vi "walidacjaTestow.vi"(11 "Odleglosci":T1[][](array[typedef]) {"Odległość [m]" format="%#.2g"}) -> (3 "Testy przeszły?":bool)   [LabVIEW 2014]
uses:
  testujPunktyVIs/Odleglosc.ctl
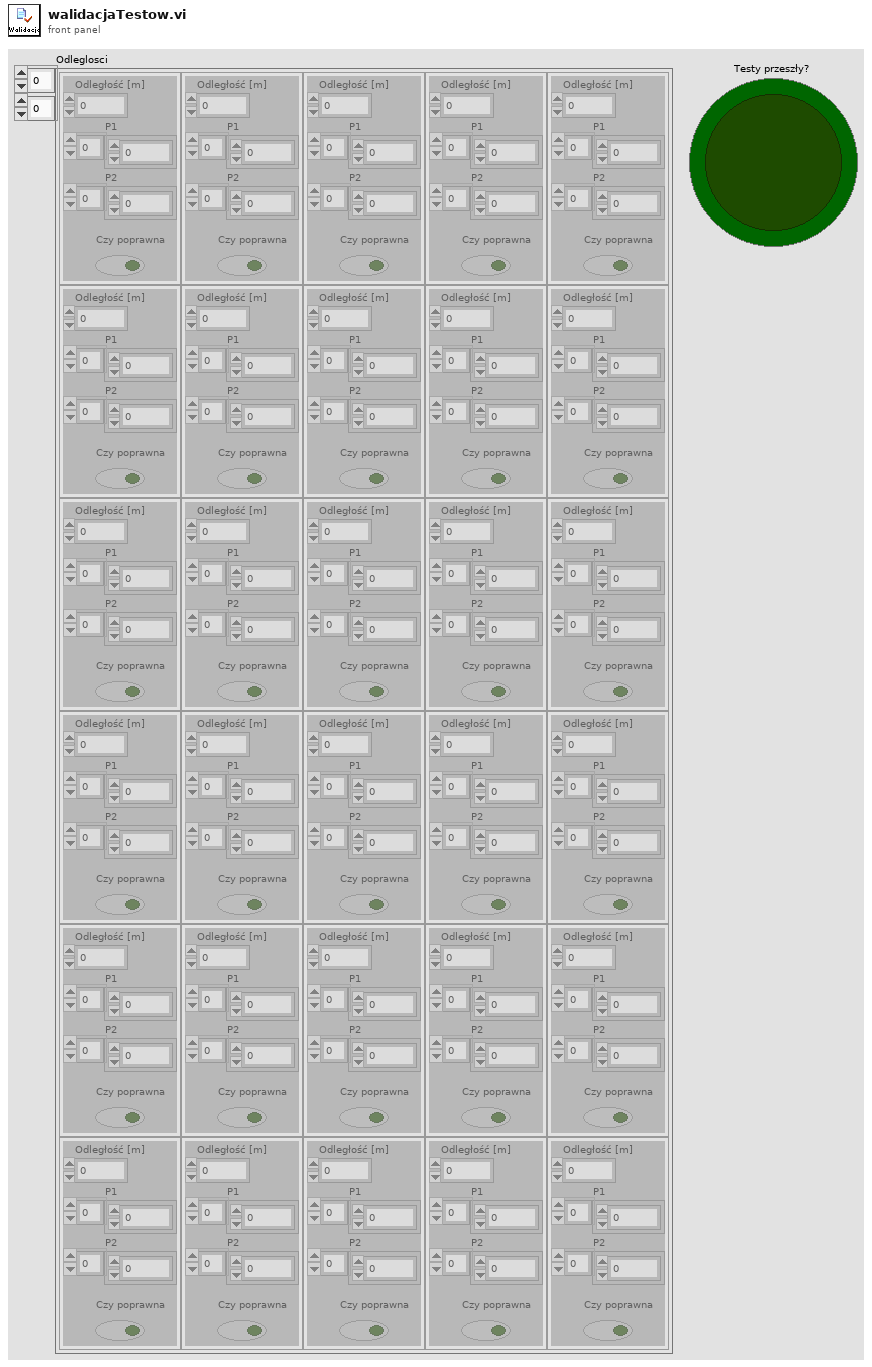
[diagram p1: front panel]
types:
  T1 = typedef "Odleglosc.ctl" = cluster{"Odległość [m]":dbl, "P1":i32[], "P2":i32[], "Czy poprawna":bool}
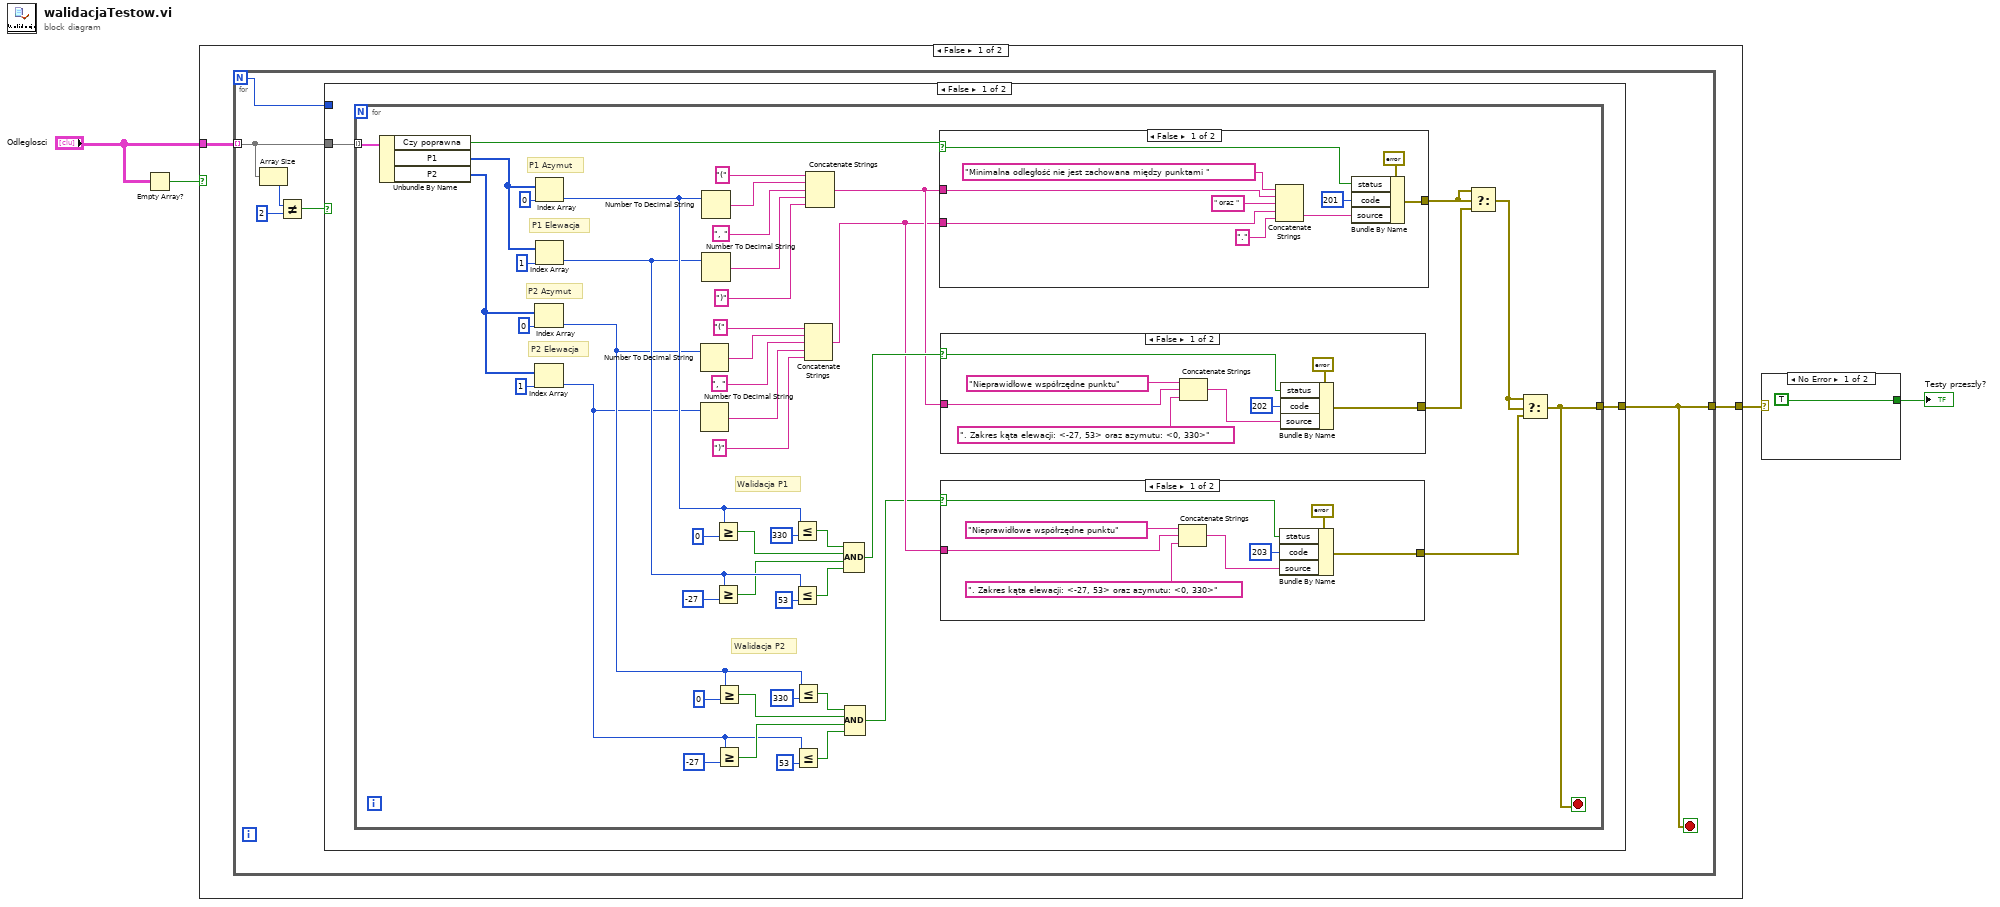
[diagram p0: block diagram]
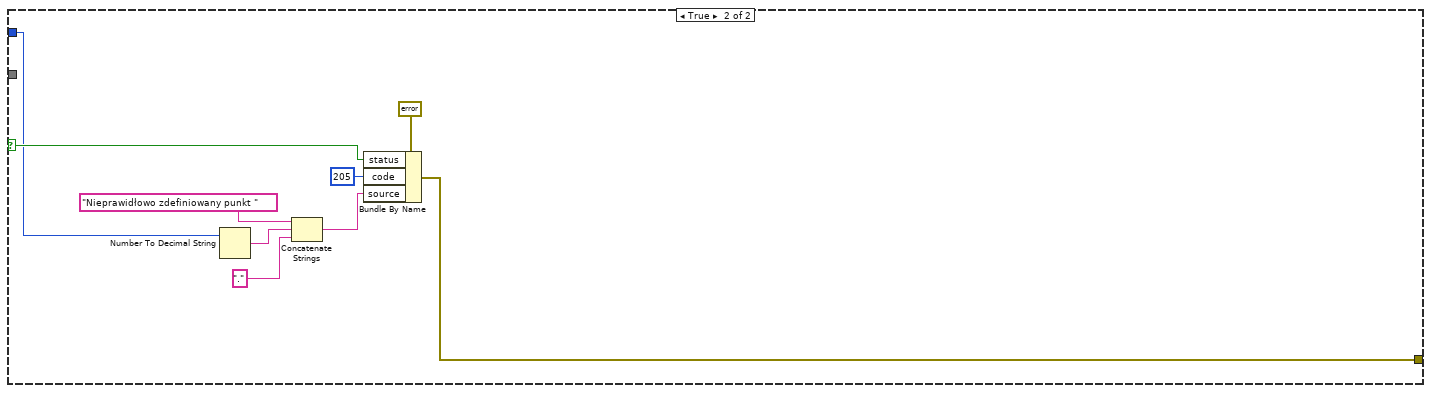
[diagram p5: hidden frame]
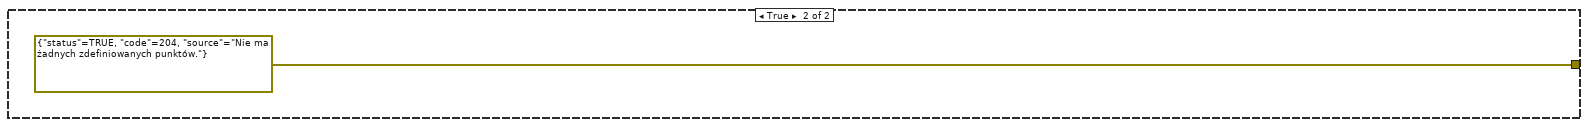
[diagram p6: hidden frame]
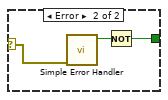
[diagram p7: hidden frame]
diagram:
  n1 = Empty Array?(array="Odleglosci") -> (empty?=w1:bool)
  n2 = case shown="False" w1 {
    tunnel: "Odleglosci" -> [w6 _]
    tunnel: [w5 errorcluster {"status"=TRUE, "code"=204, "source"="Nie ma żadnych zdefiniowanych punktów."} ("error in (no error)")] -> w4
    frame False {
      n3 = for {
        N -> [w7]
        tunnel: w6 -> [w11] mode=indexing
        tunnel: [w12] -> w5
        stop <- w12 stop-if-true
        n4 = Array Size(array=w11) -> (size(s)=w10:i32)
        n5 = Not Equal?(x=w10, y=2) -> (x != y?=w8:bool)
        n6 = case shown="False" w8 {
          selector: w8 -> [_ w95]
          tunnel: w11 -> [w14 _]
          tunnel: [w13 w89] -> w12
          tunnel: w7 -> [_ w91]
          frame False {
            n7 = for {
              tunnel: w14 -> [w61] mode=indexing
              tunnel: [w15] -> w13
              stop <- w15 stop-if-true
              # "Walidacja P2"
              # "Walidacja P1"
              # "P2 Elewacja"
              # "P2 Azymut"
              # "P1 Elewacja"
              # "P1 Azymut"
              n8 = Unbundle By Name(w61) -> ("Czy poprawna"=w60:bool, "P1"=w57:i32[], "P2"=w54:i32[])
              n9 = Index Array(array=w54, index=0) -> (element=w25:i32)
              n10 = Index Array(array=w54, index=1) -> (element=w24:i32)
              n11 = Index Array(array=w57, index=0) -> (element=w42:i32)
              n12 = Index Array(array=w57, index=1) -> (element=w38:i32)
              n13 = Number To Decimal String(number=w25) -> (decimal integer string=w44:string)  [unwired: 1 in]
              n14 = Number To Decimal String(number=w24) -> (decimal integer string=w46:string)  [unwired: 1 in]
              n15 = Number To Decimal String(number=w42) -> (decimal integer string=w49:string)  [unwired: 1 in]
              n16 = Number To Decimal String(number=w38) -> (decimal integer string=w51:string)  [unwired: 1 in]
              n17 = Greater Or Equal?(x=w42, y=0) -> (x >= y?=w36:bool)
              n18 = Greater Or Equal?(x=w38, y=-27) -> (x >= y?=w35:bool)
              n19 = Greater Or Equal?(x=w25, y=0) -> (x >= y?=w28:bool)
              n20 = Greater Or Equal?(x=w24, y=-27) -> (x >= y?=w27:bool)
              n21 = Less Or Equal?(x=w42, y=330) -> (x <= y?=w37:bool)
              n22 = Less Or Equal?(x=w38, y=53) -> (x <= y?=w34:bool)
              n23 = Less Or Equal?(x=w25, y=330) -> (x <= y?=w29:bool)
              n24 = Less Or Equal?(x=w24, y=53) -> (x <= y?=w26:bool)
              n25 = Concatenate Strings("(", w44, ", ", w46, ")") -> (w21:string)
              n26 = Concatenate Strings("(", w49, ", ", w51, ")") -> (w22:string)
              n27 = Compound Arithmetic op=AND(w37, w36, w35, w34) -> (w23:bool)
              n28 = Compound Arithmetic op=AND(w29, w28, w27, w26) -> (w20:bool)
              n29 = case shown="False" w60 {
                selector: w60 -> [w86 _]
                tunnel: w22 -> [w83 _]
                tunnel: w21 -> [w81 _]
                tunnel: [w78 _] -> w19
                frame False {
                  n30 = Concatenate Strings("Minimalna odległość nie jest zachowana między punktami " ("source"), w83, " oraz " ("string"), w81, "." ("string")) -> (w79:string)
                  n31 = Bundle By Name(cluster=errorcluster {"status"=FALSE, "code"=0, "source"=""} ("error in (no error)"), "status"=w86, "code"=201, "source"=w79) -> (w78:errorcluster)
                }
                frame True {
                }
              }
              n32 = case shown="False" w23 {
                selector: w23 -> [w71 _]
                tunnel: w22 -> [w76 _]
                tunnel: [w70 _] -> w18
                frame False {
                  n33 = Concatenate Strings("Nieprawidłowe współrzędne punktu", w76, ". Zakres kąta elewacji: <-27, 53> oraz azymutu: <0, 330>" ("string")) -> (w72:string)
                  n34 = Bundle By Name(cluster=errorcluster {"status"=FALSE, "code"=0, "source"=""} ("error in (no error)"), "status"=w71, "code"=202, "source"=w72) -> (w70:errorcluster)
                }
                frame True {
                }
              }
              n35 = case shown="False" w20 {
                selector: w20 -> [w64 _]
                tunnel: w21 -> [w68 _]
                tunnel: [w63 _] -> w16
                frame False {
                  n36 = Concatenate Strings("Nieprawidłowe współrzędne punktu", w68, ". Zakres kąta elewacji: <-27, 53> oraz azymutu: <0, 330>" ("string")) -> (w65:string)
                  n37 = Bundle By Name(cluster=errorcluster {"status"=FALSE, "code"=0, "source"=""} ("error in (no error)"), "status"=w64, "code"=203, "source"=w65) -> (w63:errorcluster)
                }
                frame True {
                }
              }
              n38 = Select(t=w19, s=w19, f=w18) -> (s? t:f=w17:errorcluster)
              n39 = Select(t=w17, s=w17, f=w16) -> (s? t:f=w15:errorcluster)
            }
          }
          frame True {
            n40 = Number To Decimal String(number=w91) -> (decimal integer string=w90:string)  [unwired: 1 in]
            n41 = Concatenate Strings("Nieprawidłowo zdefiniowany punkt " ("string"), w90, "." ("string")) -> (w93:string)
            n42 = Bundle By Name(cluster=errorcluster {"status"=TRUE, "code"=205, "source"="Nie"} ("error in (no error)"), "status"=w95, "code"=205, "source"=w93) -> (w89:errorcluster)
          }
        }
      }
    }
    frame True {
    }
  }
  n43 = case shown="No Error" w4 {
    selector: w4 -> [_ w101]
    tunnel: [TRUE w99] -> w3
    frame No Error {
    }
    frame Error {
      n44 = call <vilib>:"Simple Error Handler.vi"("error in (no error)"=w101) -> ("error?"=w100:bool)  [unwired: 4 in, 4 out]
      n45 = Not(x=w100) -> (.not. x?=w99:bool)
    }
  }
  "Testy przeszły?" <- w3
